vi "Main.vi"() -> ()   [LabVIEW 2020]
uses:
  <vilib>/DAQmx/create/channels.llb/DAQmx Create Channel (DO-Digital Output).vi
panel:
  in  "Turn on: 1\nTurn off: 0":bool
  in  "Tube":u8
  in  "Clear Pin":tag="Dev1/port0/line0:7"
  in  "Sync Pin":tag="Dev1/port0/line0:7"
  in  "Data Pin":tag="Dev1/port0/line0:7"
  in  "Write Pin":tag="Dev1/port0/line0:7"
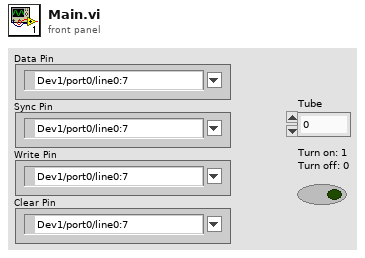
[diagram p1: front panel]
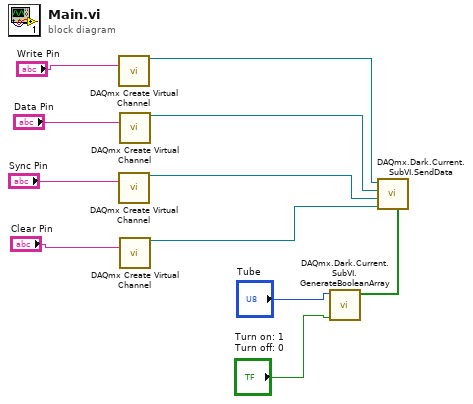
[diagram p0: block diagram]
diagram:
  n1 = call-poly <vilib>:"DAQmx Create Virtual Channel.vi"("lines"="Write Pin") -> ("task out"=w7:refnum<k21>)  [unwired: 13 in, 1 out]
  n2 = call-poly <vilib>:"DAQmx Create Virtual Channel.vi"("lines"="Sync Pin") -> ("task out"=w5:refnum<k21>)  [unwired: 13 in, 1 out]
  n3 = call-poly <vilib>:"DAQmx Create Virtual Channel.vi"("lines"="Data Pin") -> ("task out"=w6:refnum<k21>)  [unwired: 13 in, 1 out]
  n4 = call-poly <vilib>:"DAQmx Create Virtual Channel.vi"("lines"="Clear Pin") -> ("task out"=w4:refnum<k21>)  [unwired: 13 in, 1 out]
  n5 = call "DAQmx.Dark.Current.SubVI.GenerateBooleanArray.vi"("Activate: 1\nDeactivate: 0"="Turn on: 1\nTurn off: 0", "Tube"="Tube") -> ("Boolean array"=w2:bool[])  [unwired: 9 in]
  n6 = call "DAQmx.Dark.Current.SubVI.SendData.vi"("Write Pin Task In"=w7, "Data Pin Task In"=w6, "Sync Pin Task In"=w5, "Clear Pin Task In"=w4, "Data"=w2) -> ()  [unwired: 2 in, 3 out]
